vi "CS SQL Server.thread.vi"(0 "connection ID":refnum<k5>) -> ()   [LabVIEW 2014, in "CS SQL Server.lvlib"]
doc: "SQL-Server process."
uses:
  CS SQL Server.lvlib
  CS SQL Server Output Cluster.ctl
panel:
  in  "Client name":string
  in  "Data Cluster":T1 {"SQL Input Cluster"."Version" format="%.2f"}
  in  "stop":bool
  in  "SQL Read Output":T2
  in  "SQL Read Input":T3 {"Version" format="%.2f"}
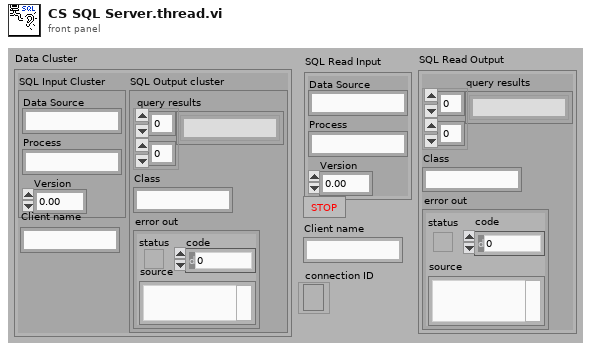
[diagram p1: front panel]
types:
  T1 = cluster{"SQL Input Cluster":cluster{"Data Source":string, "Process":string, "Version":dbl}, "SQL Output cluster":cluster{"query results":string[][], "Class":string, "error out":errorcluster}, "Client name":string}
  T2 = typedef "CS SQL Server.lvlib/CS SQL Server Output Cluster.ctl" = cluster{"query results":string[][], "Class":string, "error out":errorcluster}
  T3 = cluster{"Data Source":string, "Process":string, "Version":dbl}
  T4 = enum16{"add connection", "remove connection", "kill all connections", "default"}
  T5 = cluster{"SQL Read Input":cluster{"Data Source":string, "Process":string, "Version":dbl}, "SQL Read Output":T2, "Client name":string}
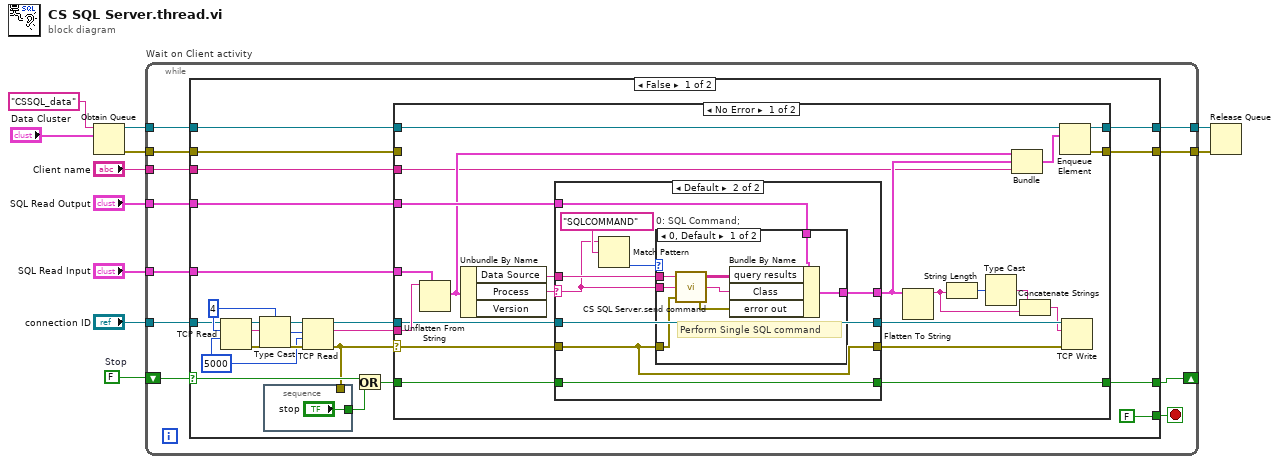
[diagram p0: block diagram]
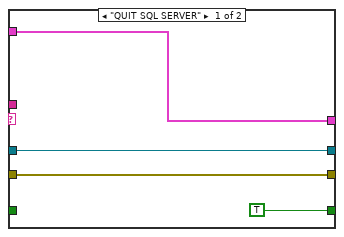
[diagram p2: hidden frame]
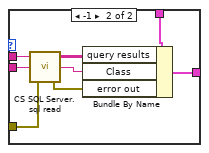
[diagram p3: hidden frame]
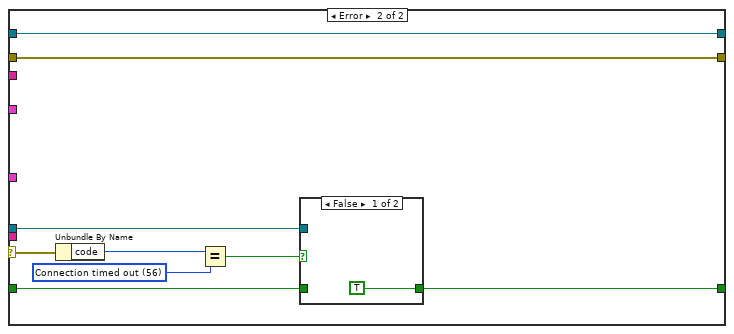
[diagram p4: hidden frame]
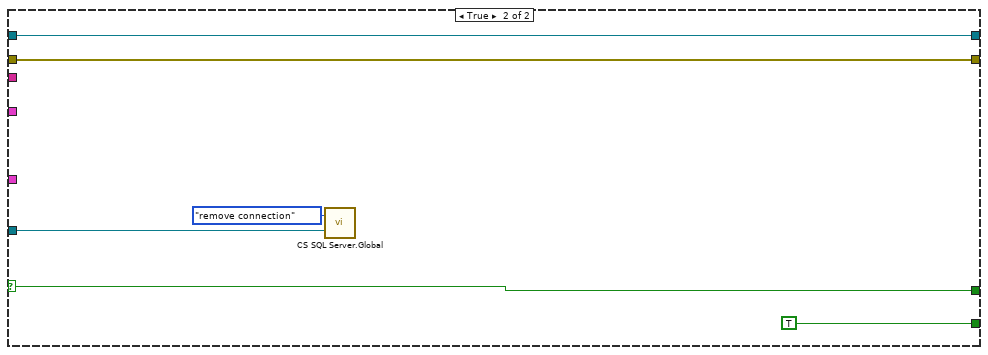
[diagram p6: hidden frame]
diagram:
  w4 = FALSE  # Stop
  n1 = Obtain Queue(name (unnamed)="CSSQL_data", element data type="Data Cluster") -> (queue out=w11:refnum<queue>, error out=w8:errorcluster)  [unwired: 3 in, 1 out]
  n2 = while "Wait on Client activity" {
    tunnel: "connection ID" -> [w22]
    tunnel: w11 -> [w21]
    tunnel: [w20] -> w10
    tunnel: [w19] -> w9
    tunnel: w8 -> [w18]
    shift-right: [w16] -> _
    shift-left: w4 -> [w17]
    tunnel: "Client name" -> [w14]
    tunnel: "SQL Read Output" -> [w13]
    tunnel: "SQL Read Input" -> [w12]
    stop <- w15 stop-if-true
    n3 = case shown="False" w17 {
      selector: w17 -> [w28 w113]
      tunnel: w22 -> [w38 w109]
      tunnel: w21 -> [w36 w111]
      tunnel: [w35 w111] -> w20
      tunnel: [w34 w110] -> w19
      tunnel: w18 -> [w33 w110]
      tunnel: [w31 w113] -> w16
      tunnel: [FALSE TRUE] -> w15
      tunnel: w14 -> [w25 _]
      tunnel: w13 -> [w24 _]
      tunnel: w12 -> [w23 _]
      frame False {
        w37 = 5000
        w44 = 4
        n4 = TCP Read(connection ID=w38, bytes to read=w44, 9:w37) -> (connection ID out=w41:refnum<k5>, data out=w43:string, error out=w40:errorcluster)  [unwired: 2 in]
        n5 = Type Cast(type=w44, x=w43) -> (*(type *) &x=w42:i32)
        n6 = TCP Read(connection ID=w41, bytes to read=w42, error in (no error)=w40, 9:w37) -> (connection ID out=w32:refnum<k5>, data out=w39:string, error out=w26:errorcluster)  [unwired: 1 in]
        n7 = stacked-sequence {
          tunnel: ["stop"] -> w29
          tunnel: w26 -> [_]
          frame #0 {
          }
        }
        n8 = Or(x=w28, y=w29) -> (x .or. y?=w27:bool)
        n9 = case shown="No Error" w26 {
          selector: w26 -> [w58 w101]
          tunnel: w23 -> [w62 _]
          tunnel: w24 -> [w61 _]
          tunnel: w39 -> [w67 _]
          tunnel: w32 -> [w66 w102]
          tunnel: w36 -> [w65 w100]
          tunnel: [w64 w100] -> w35
          tunnel: [w63 w99] -> w34
          tunnel: w33 -> [_ w99]
          tunnel: w27 -> [w57 w98]
          tunnel: [w56 w97] -> w31
          tunnel: w25 -> [w46 _]
          frame No Error {
            n10 = Unflatten From String(type=w62, binary string=w67) -> (value=w60:T3)  [unwired: 3 in, 2 out]
            n11 = Unbundle By Name(w60) -> ("Data Source"=w48:string, "Process"=w47:string)  [unwired: 1 out]
            n12 = case shown="Default" w47 {
              selector: w47 -> [_ w73]
              tunnel: w66 -> [w70 w78]
              tunnel: w61 -> [w68 w80]
              tunnel: w58 -> [w69 w75]
              tunnel: w57 -> [_ w79]
              tunnel: [TRUE w79] -> w56
              tunnel: [w69 w75] -> w55
              tunnel: [w70 w78] -> w54
              tunnel: [w68 w77] -> w49
              tunnel: w48 -> [_ w76]
              frame "QUIT SQL SERVER" {
              }
              frame Default {
                n13 = Match Pattern(string=w73, regular expression="SQLCOMMAND") -> (offset past match=w72:i32)  [unwired: 1 in, 3 out]
                n14 = case "0: SQL Command;" shown="0, Default" w72 {
                  tunnel: w80 -> [w83 w93]
                  tunnel: [w82 w92] -> w77
                  tunnel: w76 -> [w84 w91]
                  tunnel: w73 -> [w81 w90]
                  tunnel: w75 -> [w85 w89]
                  frame 0, Default {
                    # "Perform Single SQL command"
                    n15 = call "CS SQL Server.send command.vi"("error in (no error)"=w85, "SQL Command"=w81, "Data Source"=w84) -> ("error out"=w86:errorcluster, "Class"=w87:string, "query results"=w88:string[][])
                    n16 = Bundle By Name(cluster=w83, "query results"=w88, "Class"=w87, "error out"=w86) -> (w82:T2)
                  }
                  frame -1 {
                    n17 = call "CS SQL Server.sql read.vi"("error in (no error)"=w89, "object"=w90, "Data Source"=w91) -> ("error out"=w94:errorcluster, "Class"=w96:string, "query results"=w95:string[][])
                    n18 = Bundle By Name(cluster=w93, "query results"=w95, "Class"=w96, "error out"=w94) -> (w92:T2)
                  }
                }
              }
            }
            n19 = Flatten To String(anything=w49) -> (data string=w53:string)  [unwired: 3 in, 2 out]
            n20 = String Length(string=w53) -> (length=w51:i32)
            n21 = Type Cast(x=w51) -> (*(type *) &x=w52:string)  [unwired: 1 in]
            n22 = Bundle("SQL Read Input"=w60, "SQL Read Output"=w49, "Client name"=w46) -> (w59:T5)  [unwired: 1 in]
            n23 = Concatenate Strings(w52, w53) -> (w50:string)
            n24 = Enqueue Element(queue=w65, element=w59) -> (queue out=w64:refnum<queue>, error out=w63:errorcluster)  [unwired: 2 in, 1 out]
            n25 = TCP Write(connection ID=w54, data in=w50, error in (no error)=w55) -> ()  [unwired: 1 in, 3 out]
          }
          frame Error {
            w104 = 56 items=["No Error", "Argument Error", "Memory Full", "Out of Zone", "End of File", "File Already Open", "Generic File IO Error", "File Not Found", "File Permission Error", "Disk Full", "Duplicate Path", "Too Many Files Open", "Not Enabled", "Resource File Not Found", "Cannot Add Resource", "Resource Not Found", "Image Not Found", "Image Memory Error", "Pen Does Not Exist", "Config Bad Type", "Config Token Not Found", "Config Parse Error", "Config Memory Error", "Bad External Code Format", "Bad External Code Offset", "External Code Not Present", "Null Window", "Destroy Window Mixup", "Null Menu", "Print Aborted", "Bad Print Record", "Print Driver Error", "Windows Error During Print", "Memory Error During Print", "Print Dialog Error", "Generic Print Error", "Invalid Device Refnum", "Device Not Found", "Device Parameter Error", "Device Unit Error", "Can't Open Device", "Device Call Aborted", "Generic Error", "Cancelled By User", "Object ID Too Low", "Object ID Too High", "Object Not In Heap", "Unknown Heap", "Bad DefProc ID", "DefProc Not In Table", "Message Out Of Range", "Null Method", "Unknown Message", "Manager Call Not Supported", "Bad address", "Connection In progress", "Connection timed out", "Connection is already in progress", "Network attribute not supported", "Network error", "Address in use", "System out of memory", "Connection aborted", "Connection refused", "Connection is not connected", "Connection is already connected", "Connection closed", "Initialize error (interapplication manager)", "Bad occurrence", "Wait on unbound occurrence handler", "Occurrence queue overflow", "Bad path", "Semaphore not signaled", "Unrecognized type (interapplication manager)"] ("1st Error to Convert")
            n26 = Unbundle By Name(w101) -> ("code"=w103:i32)
            n27 = Equal?(x=w103, y=w104) -> (x = y?=w105:bool)
            n28 = case shown="False" w105 {
              tunnel: w102 -> [_ _]
              tunnel: w98 -> [_ w107]
              tunnel: [TRUE w107] -> w97
              frame False {
              }
              frame True {
              }
            }
          }
        }
      }
      frame True {
        n29 = call "CS SQL Server.Global.vi"("command"=T4."remove connection", "connection"=w109) -> ()  [unwired: 17 in, 1 out]
      }
    }
  }
  n30 = Release Queue(queue=w10, error in (no error)=w9) -> ()  [unwired: 1 in, 3 out]
